vi "diffrerential array.vi"(11 "Array in":dbl[](array[numeric])) -> (3 "Array":dbl[](array[numeric]))   [LabVIEW 2024]
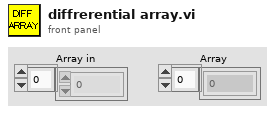
[diagram p1: front panel]
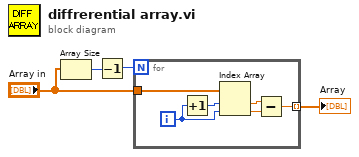
[diagram p0: block diagram]
diagram:
  n1 = Array Size(array="Array in") -> (size(s)=w4:i32)
  n2 = Decrement(x=w4) -> (x-1=w3:i32)
  n3 = for {
    N: w3 -> [_]
    tunnel: "Array in" -> [w8]
    tunnel: [w5] -> w2 mode=indexing
    i -> [w9]
    n4 = Increment(x=w9) -> (x+1=w10:i32)
    n5 = Index Array(array=w8, index #1=w10, index #2=w9) -> (element #1=w6:dbl, element #2=w7:dbl)
    n6 = Subtract(x=w6, y=w7) -> (x-y=w5:dbl)
  }
  "Array" <- w2
